vi "DBLayerGen.vi"(6 "Layer":u32=160, 10 "HatchPow":T5={"Power"=300.0, "Mark Speed"=400.0, "Jump Speed"=1000.0}, 11 "RectHatch":T6={"Width"=10.0, "Height"=10.0, "Angle"=45.0, "OffX"=0.1, "OffY"=0.1, "Spacing"=0.1} {"Spacing" format="%#_13g"; "OffY" format="%#_13g"; "OffX" format="%#_13g"; "Height" format="%#_13g"; "Width" format="%#_13g"}) -> (3 "PathSups":T1[](array[typedef]))   [LabVIEW 2014]
uses:
  TypeDefs/RectHatch.ctl
  TypeDefs/PowerSpeed.ctl
  TypeDefs/PathSupreme.ctl
  PSup2SCAN/Sub/VelocityProfile.ctl
  PSup2SCAN/Sub/PathCut.ctl
  PSup2SCAN/Sub/Segment.ctl
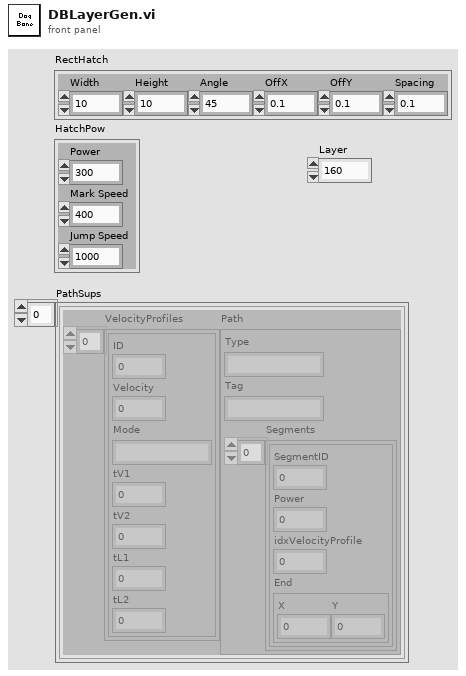
[diagram p1: front panel]
types:
  T1 = typedef "PathSupreme.ctl" = cluster{"VelocityProfiles":T2[], "Path":T3}
  T2 = typedef "VelocityProfile.ctl" = cluster{"ID":u32, "Velocity":dbl, "Mode":string, "tV1":u32, "tV2":u32, "tL1":u32, "tL2":u32}
  T3 = typedef "PathCut.ctl" = cluster{"Type":string, "Tag":string, "Segments":T4[]}
  T4 = typedef "Segment.ctl" = cluster{"SegmentID":u16, "Power":sgl, "idxVelocityProfile":u16, "End":cluster{"X":sgl, "Y":sgl}}
  T5 = typedef "PowerSpeed.ctl" = cluster{"Power":dbl, "Mark Speed":dbl, "Jump Speed":dbl}
  T6 = typedef "RectHatch.ctl" = cluster{"Width":dbl, "Height":dbl, "Angle":sgl, "OffX":dbl, "OffY":dbl, "Spacing":dbl}
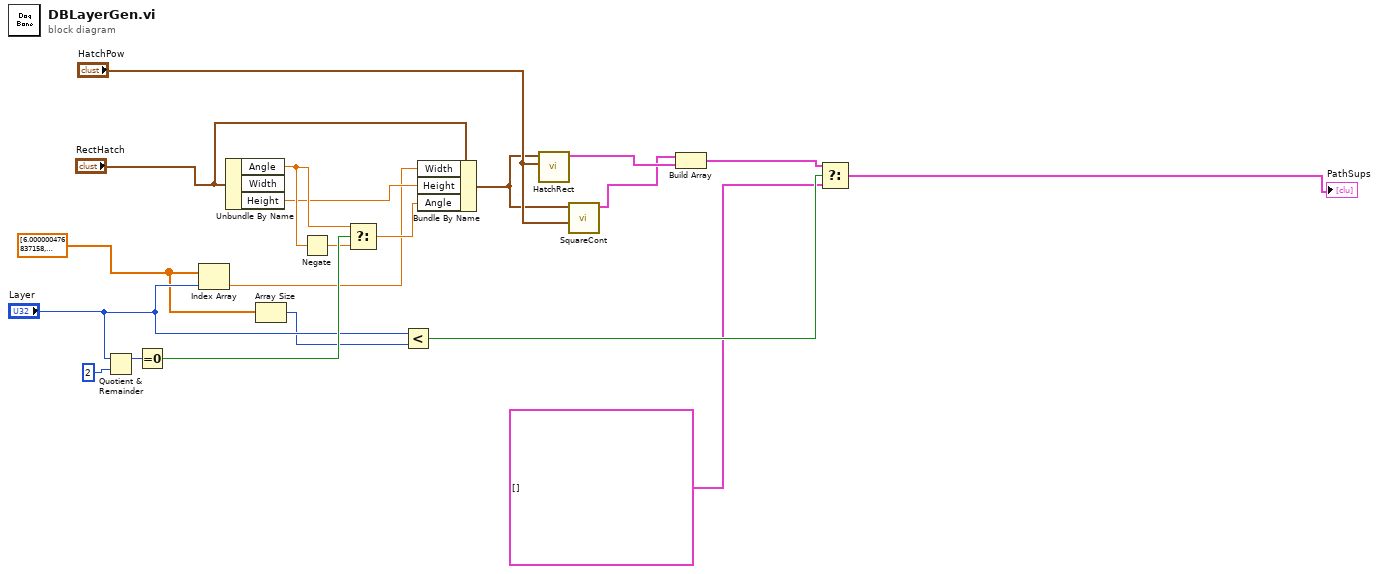
[diagram p0: block diagram]
diagram:
  w1 = dbl[] [6.000000476837158, 5.999999523162842, 5.999999523162842, 6.000000476837158, 6.000000476837158, 5.999999523162842, 5.999999523162842, 6.000000476837158, 6.000000476837158, 5.999999523162842, 5.999999523162842, 6.000000476837158, 6.000000476837158, 5.999999523162842, 5.999999523162842, 6.000000476837158, 6.000000476837158, 5.999999523162842, 5.999999523162842, 6.000000476837158, 6.000000476837158, 6.000000476837158, 5.999999523162842, 5.999999523162842, 5.999999523162842, 6.000000476837158, 6.000000476837158, 5.999999523162842, 5.999999523162842, 6.000000476837158, 6.000000476837158, 5.999999523162842, 5.999999523162842, 6.000000476837158, 6.000000476837158, 5.999999523162842, 5.999999523162842, 6.000000476837158, 6.000000476837158, 5.999999523162842, 5.999999523162842, 6.000000476837158, 6.000000476837158, 5.999999523162842, 5.971573352813721, 5.971574306488037, 5.7715744972229, 5.771573543548584, 5.571572780609131, 5.571573734283447, 5.3715739250183105, 5.371572971343994, 5.171573162078857, 5.171574115753174, 4.971574306488037, 4.971573352813721, 4.771573066711426, 4.771574020385742, 4.571573734283447, 4.571573257446289, 4.371572971343994, 4.371573448181152, 4.171573638916016, 4.171573162078857, 3.9715733528137207, 3.971573829650879, 3.771573543548584, 3.771573066711426, 3.571573257446289, 3.5715737342834473, 3.3715734481811523, 3.371572971343994, 3.1715731620788574, 3.1715736389160156, 2.971573829650879, 2.9715733528137207, 2.7715728282928467, 2.771573543548584, 2.5715737342834473, 2.57157301902771, 2.371572732925415, 2.3715732097625732, 2.1715734004974365, 2.1715729236602783, 1.9715731143951416, 1.9715735912322998, 1.7715733051300049, 1.7715728282928467, 1.5736470222473145, 1.5736474990844727, 1.4028316736221313, 1.4028311967849731, 1.2743767499923706, 1.2743772268295288, 1.17326021194458, 1.1732598543167114, 1.0935570001602173, 1.0935577154159546, 1.0455418825149536, 1.045541524887085, 1.0157402753829956, 1.0157405138015747, 1.0000001192092896, 1.0000001192092896, 0.9999998807907104, 0.9999998807907104, 0.9999998807907104, 1.0000001192092896, 1.0000001192092896, 0.9999998807907104, 0.9999998807907104, 1.0000001192092896, 1.0000001192092896, 0.9999998807907104, 0.9999999403953552, 1.0000001192092896, 1.0, 0.9999999403953552, 0.9999999403953552, 1.0, 1.0, 0.9999999403953552, 0.9999999403953552, 1.0, 1.0, 0.9999999403953552, 0.9999999403953552, 1.0, 1.0, 0.9999999403953552, 1.0, 1.0, 1.0, 1.0, 1.0, 0.9999999403953552, 0.9999999403953552, 1.0, 1.0, 0.9999999403953552, 0.9999999403953552, 1.0, 1.0, 0.9999999403953552, 0.9999999403953552, 1.0, 1.0, 0.9999998807907104, 0.9999998807907104, 1.0, 1.0000001192092896, 0.9999998807907104, 0.9999998807907104, 1.0000001192092896, 1.0000001192092896, 0.9999998807907104, 0.9999998807907104, 1.0000001192092896, 1.0000001192092896, 0.9999998211860657, 0.9999998211860657, 1.0000001192092896, 1.0000001192092896, 0.9999998211860657, 0.9999998211860657, 1.0000001192092896, 1.0000001192092896, 0.9999998211860657, 0.9999997615814209, 1.0000001192092896, 1.0000001192092896, 0.9999997615814209, 0.9999997615814209, 1.0000001192092896, 1.000000238418579, 0.9999997615814209, 0.9999997615814209, 1.000000238418579, 1.000000238418579, 0.9999997615814209, 0.9999997019767761, 1.000000238418579, 1.000000238418579, 0.9999997019767761, 0.9999997019767761, 1.000000238418579, 1.0157405138015747, 1.0157400369644165, 1.0455412864685059, 1.045541524887085, 1.0935571193695068, 1.0935571193695068, 1.1732593774795532, 1.1732597351074219, 1.2743765115737915, 1.2743759155273438, 1.4028310775756836, 1.4028315544128418, 1.5736459493637085, 1.5736454725265503, 1.7715709209442139, 1.771571397781372, 1.9715718030929565, 1.9715712070465088, 2.1715710163116455, 2.171571731567383, 2.3715715408325195, 2.3715708255767822, 2.571571111679077, 2.5715718269348145, 2.771571636199951, 2.771570920944214, 2.971571445465088, 2.971572160720825, 3.171571969985962, 3.1715712547302246, 3.3715710639953613, 3.3715717792510986, 3.5715715885162354, 3.571570873260498, 3.771571636199951, 3.7715723514556885, 3.971572160720825, 3.971571445465088, 4.171571254730225, 4.171572208404541, 4.371572017669678, 4.371571063995361, 4.571570873260498, 4.5715718269348145, 4.771572589874268, 4.771571636199951, 4.971571445465088, 4.971572399139404, 5.171572208404541, 5.171571254730225, 5.371571063995361, 5.371572017669678, 5.5715718269348145, 5.571570873260498, 5.771571636199951, 5.771572589874268, 5.971572399139404, 5.971571445465088, 5.999999523162842, 6.000000476837158, 6.000000476837158, 5.999999523162842, 5.999999523162842, 6.000000476837158, 6.000000476837158, 5.999999523162842, 5.999999523162842, 6.000000476837158, 6.000000476837158, 5.999999523162842, 5.999999523162842, 6.000000476837158, 6.000000476837158, 5.999999523162842, 5.999999523162842, 6.000000476837158, 6.000000476837158, 5.999999523162842, 5.999999523162842, 6.000000476837158] ("DogWidths")
  n1 = Quotient & Remainder(x="Layer", y=u8 2) -> (x-y*floor(x/y)=w20:u32)  [unwired: 1 out]
  n2 = Equal To 0?(x=w20) -> (x = 0?=w18:bool)
  n3 = Index Array(array=w1, index="Layer") -> (element=w8:dbl)
  n4 = Unbundle By Name("RectHatch") -> ("Angle"=w14:sgl, "Height"=w11:dbl)  [unwired: 1 out]
  n5 = Array Size(array=w1) -> (size(s)=w6:i32)
  n6 = Negate(x=w14) -> (-x=w15:sgl)
  n7 = Select(t=w14, s=w18, f=w15) -> (s? t:f=w13:sgl)
  n8 = Less?(x="Layer", y=w6) -> (x < y?=w5:bool)
  n9 = Bundle By Name(cluster="RectHatch", "Width"=w8, "Height"=w11, "Angle"=w13) -> (w12:T6)
  n10 = call "HatchRect.vi"("HatchPow"="HatchPow", "RectHatch"=w12) -> ("PathSupreme"=w10:T1)  [unwired: 9 in]
  n11 = call "SquareCont.vi"("ContPow"="HatchPow", "RectHatch"=w12) -> ("PathSupreme"=w9:T1)  [unwired: 9 in]
  n12 = Build Array(w9, w10) -> (w4:T1[])
  n13 = Select(t=w4, s=w5, f=T1[] []) -> (s? t:f=→"PathSups":T1[])
